vi "PGM.vi"(2 "baud rate (9600)":u32=115200 caption="보 전송속도(9600)", 3 "(XY00)":string, 4 "Port":refnum<visa-resource-name>="COM4" caption="VISA 리소스 이름") -> (0 "Error Out":errorcluster caption="에러 출력", 1 "VISA out":refnum<visa-resource-name>)   [LabVIEW 2010]
uses:
  <vilib>/Instr/_visa.llb/VISA Flush IO Buffer Mask.ctl
  <vilib>/Instr/_visa.llb/VISA Configure Serial Port (Instr).vi
panel:
  out "Commend Count":u32
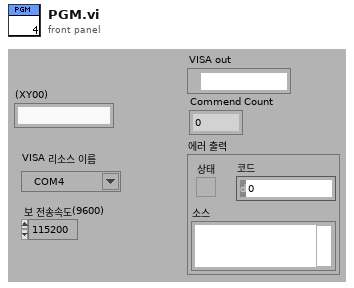
[diagram p1: front panel]
types:
  T1 = typedef "VISA Flush IO Buffer Mask.ctl" = u16
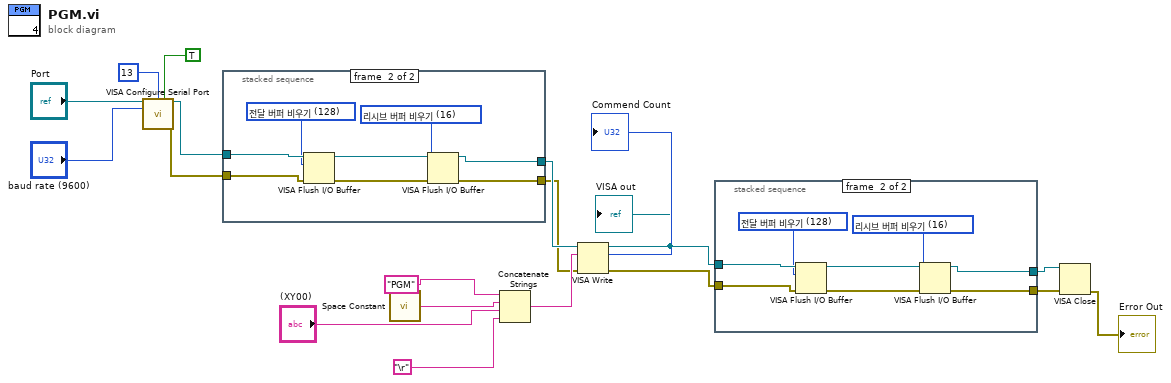
[diagram p0: block diagram]
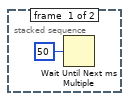
[diagram p2: hidden frame]
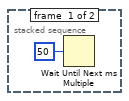
[diagram p3: hidden frame]
diagram:
  n1 = call-poly "VISA Configure Serial Port"("VISA resource name"="Port", "termination char\n(0xA = '\\n' = LF)"=i16 13 ("termination char\n(0xA = '\\n' = LF)"), "Enable Termination\nChar (T)"=TRUE ("Enable Termination\nChar (T)"), "baud rate (9600)"="baud rate (9600)") -> ("VISA resource name out"=w9:refnum<visa-resource-name>, "error out"=w8:errorcluster)  [unwired: 10 in]
  n2 = stacked-sequence {
    tunnel: w9 -> [_ w28]
    tunnel: w8 -> [_ w27]
    tunnel: [_ w23] -> w7
    tunnel: [_ w22] -> w6
    frame #0 {
      n3 = Wait Until Next ms Multiple(millisecond multiple=u32 50 ("ms 배수")) -> ()  [unwired: 1 out]
    }
    frame #1 {
      w21 = T1 16 items=["리시브 버퍼 비우기"=16, "전달 버퍼 디바이스에 쓰기"=32, "리시브 버퍼 비우기(I/O 없음)"=64, "전달 버퍼 비우기"=128] ("Mask")
      w26 = T1 128 items=["리시브 버퍼 비우기"=16, "전달 버퍼 디바이스에 쓰기"=32, "리시브 버퍼 비우기(I/O 없음)"=64, "전달 버퍼 비우기"=128] ("Mask")
      n4 = VISA Flush I/O Buffer(VISA resource name=w28, mask (16)=w26, error in (no error)=w27) -> (VISA resource name out=w25:refnum<visa-resource-name>, error out=w24:errorcluster)
      n5 = VISA Flush I/O Buffer(VISA resource name=w25, mask (16)=w21, error in (no error)=w24) -> (VISA resource name out=w23:refnum<visa-resource-name>, error out=w22:errorcluster)
    }
  }
  n6 = call <vilib>:"Space Constant.vi"() -> ("String"=w18:string)
  n7 = Concatenate Strings("PGM", w18, "(XY00)", "\r") -> (w15:string)
  n8 = VISA Write(VISA resource name=w7, write buffer=w15, error in (no error)=w6) -> (VISA resource name out=w2:refnum<visa-resource-name>, return count=→"Commend Count":u32, error out=w1:errorcluster)
  "VISA out" <- w2
  n9 = stacked-sequence {
    tunnel: w2 -> [_ w37]
    tunnel: w1 -> [_ w36]
    tunnel: [_ w32] -> w4
    tunnel: [_ w31] -> w5
    frame #0 {
      n10 = Wait Until Next ms Multiple(millisecond multiple=u32 50 ("ms 배수")) -> ()  [unwired: 1 out]
    }
    frame #1 {
      w30 = T1 16 items=["리시브 버퍼 비우기"=16, "전달 버퍼 디바이스에 쓰기"=32, "리시브 버퍼 비우기(I/O 없음)"=64, "전달 버퍼 비우기"=128] ("Mask")
      w35 = T1 128 items=["리시브 버퍼 비우기"=16, "전달 버퍼 디바이스에 쓰기"=32, "리시브 버퍼 비우기(I/O 없음)"=64, "전달 버퍼 비우기"=128] ("Mask")
      n11 = VISA Flush I/O Buffer(VISA resource name=w37, mask (16)=w35, error in (no error)=w36) -> (VISA resource name out=w34:refnum<visa-resource-name>, error out=w33:errorcluster)
      n12 = VISA Flush I/O Buffer(VISA resource name=w34, mask (16)=w30, error in (no error)=w33) -> (VISA resource name out=w32:refnum<visa-resource-name>, error out=w31:errorcluster)
    }
  }
  n13 = VISA Close(VISA resource name=w4, error in (no error)=w5) -> (error out=→"Error Out":errorcluster)
